vi "modbus asynch.vi"(11 "Modbus Module runtime in":refnum<class "Modbus Module runtime.lvclass">) -> (0 "error out":errorcluster)   [LabVIEW 2014, in "Modbus Module runtime.lvclass"]
uses:
  Modbus Module runtime.lvclass
  Modbus Module runtime.lvclass/Modbus Module runtime.ctl
  process state enum.ctl
  message to background process.ctl
  command enum.ctl
  <vilib>/NI/Tag Bus/table/data table.ctl
  response from background process.ctl
  response enum.ctl
  <vilib>/NI/Tag Bus/table/data table.lvlib
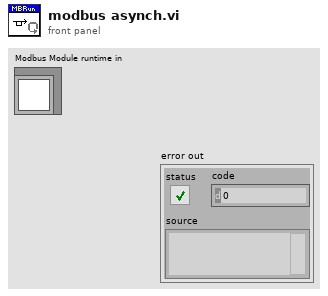
[diagram p1: front panel]
types:
  T1 = typedef "Modbus Module runtime.lvclass/response from background process.ctl" = cluster{"response enum":T2, "datapack":refnum<data-value>, "error code":i32}
  T2 = typedef "Modbus Module runtime.lvclass/response enum.ctl" = enum16{"exit", "return buffer", "error"}
  T3 = typedef "Modbus Module runtime.lvclass/message to background process.ctl" = cluster{"command enum":T4, "datapack":refnum<data-value>}
  T4 = typedef "Modbus Module runtime.lvclass/command enum.ctl" = enum16{"stop", "input", "output"}
  T5 = typedef "Modbus Module runtime.lvclass/process state enum.ctl" = enum16{"wait for message", "report error", "exit"}
  T6 = typedef "tag bus.lvlib/data table.lvlib/data table.ctl" = cluster{"Double":dbl[], "Single":sgl[], "I64":i64[], "I32":i32[], "I16":i16[], "I8":i8[], "U64":u64[], "U32":u32[], "U16":u16[], "U8":u8[], "Boolean":bool[], "String":string[], "Array of Double":cluster{"DBL Array":dbl[]}[], "Array of Single":cluster{"SGL Array":sgl[]}[], "Array of I64":cluster{"I64 Array":i64[]}[], "Array of I32":cluster{"I32 Array":i32[]}[], "Array of I16":cluster{"I16 Array":i16[]}[], "Array of I8":cluster{"I8 Array":i8[]}[], "Array of U64":cluster{"U64 Array":u64[]}[], "Array of U32":cluster{"U32 Array":u32[]}[], "Array of U16":cluster{"U16 Array":u16[]}[], "Array of U8":cluster{"U8 Array":u8[]}[], "Array of Boolean":cluster{"Boolean Array":bool[]}[], "Array of String":cluster{"String Array":string[]}[]}
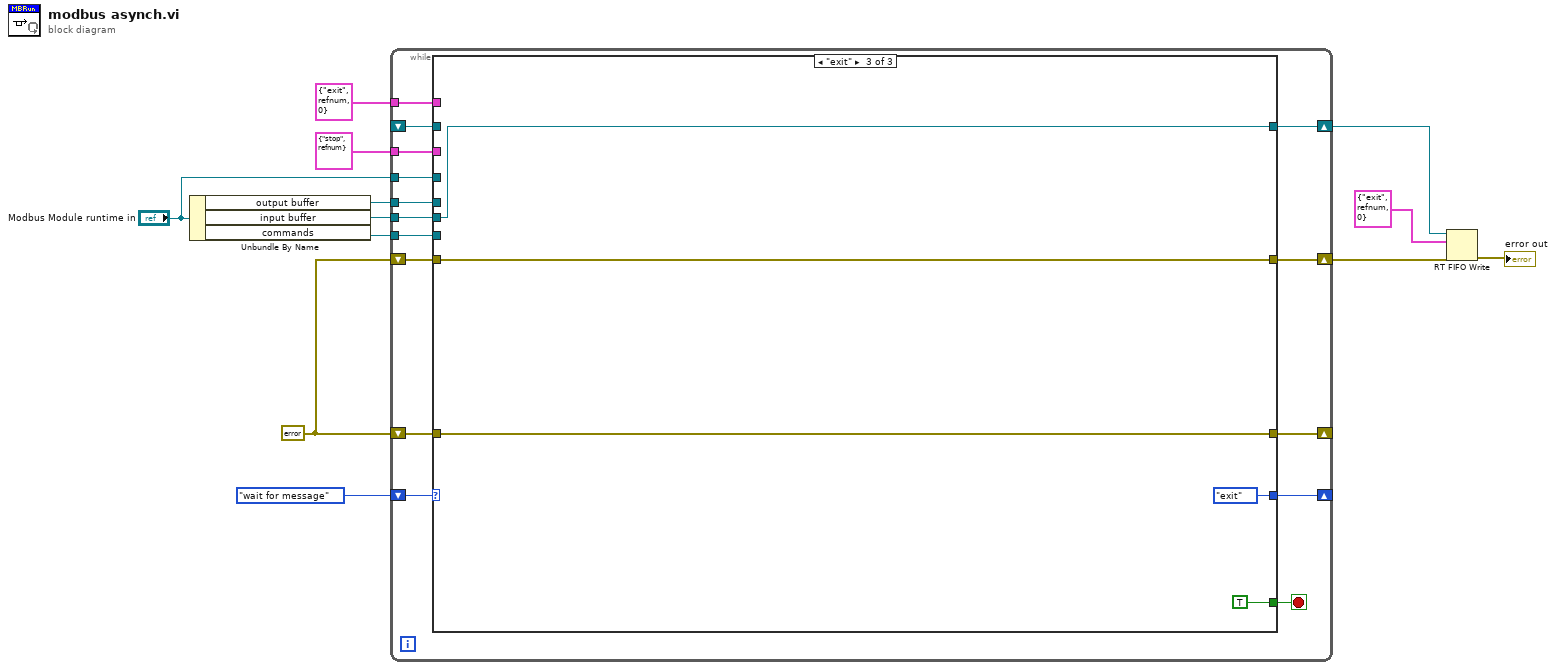
[diagram p0: block diagram]
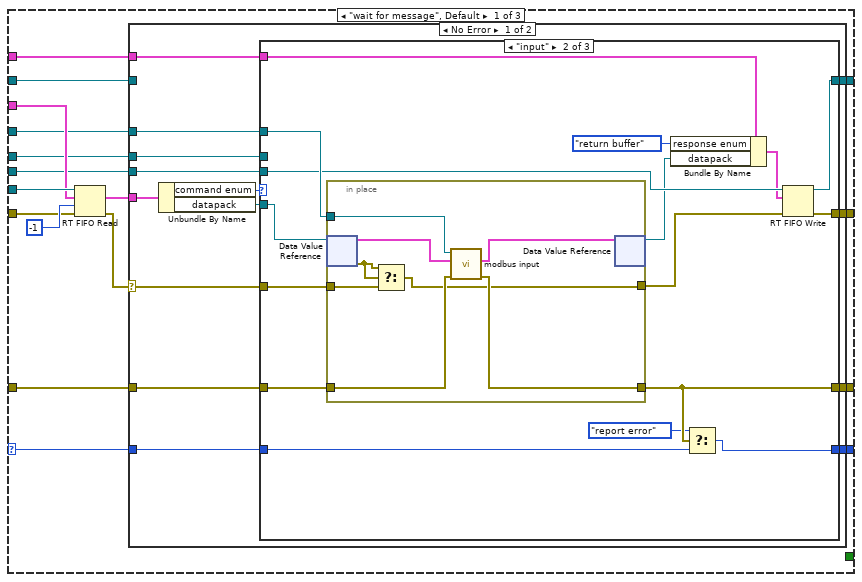
[diagram p2: hidden frame]
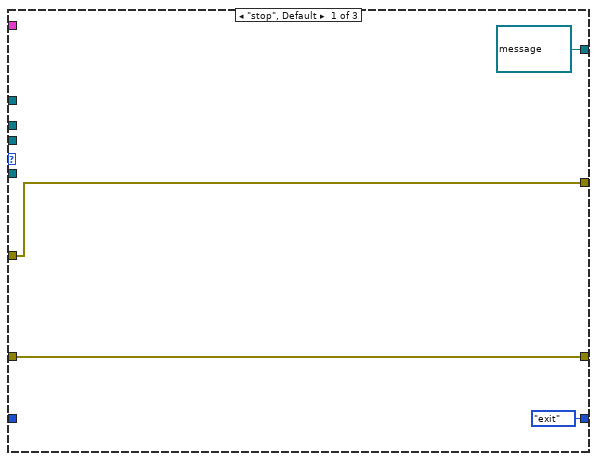
[diagram p3: hidden frame]
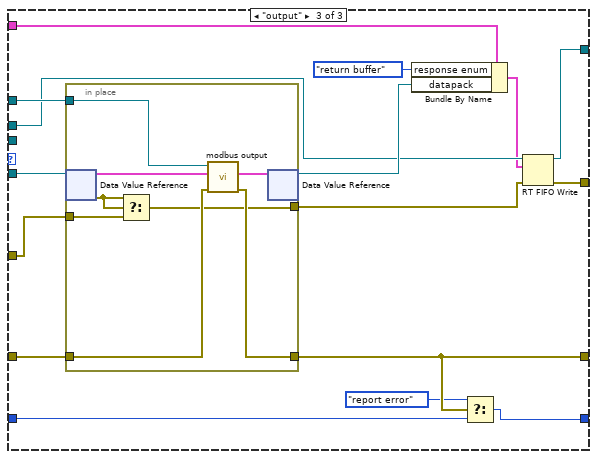
[diagram p4: hidden frame]
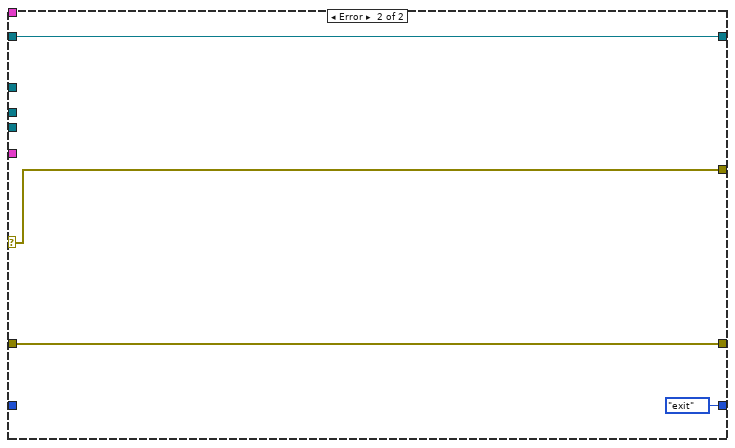
[diagram p5: hidden frame]
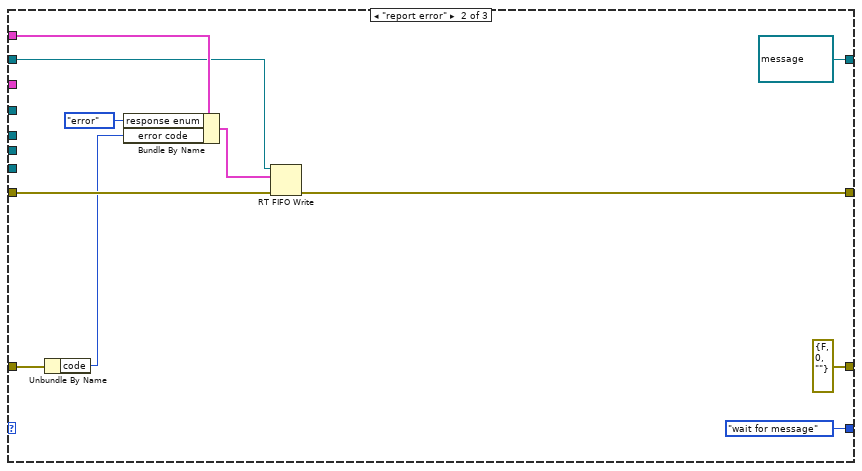
[diagram p6: hidden frame]
diagram:
  w7 = errorcluster {"status"=FALSE, "code"=0, "source"=""} ("error out")
  n1 = Unbundle By Name("Modbus Module runtime in") -> ("output buffer"=w5:refnum<k33>, "input buffer"=w8:refnum<k33>, "commands"=w11:refnum<k33>)
  n2 = while {
    shift-right: [w18] -> _
    shift-left: process_state_enum."wait for message" ("process state") -> [w27]
    tunnel: w11 -> [w26]
    tunnel: T3 {"command enum"=enum."stop", "datapack"=refnum} ("message") -> [w25]
    shift-right: [w21] -> w4
    shift-left: w7 -> [w24]
    tunnel: "Modbus Module runtime in" -> [w23]
    tunnel: w8 -> [w22]
    shift-right: [w19] -> _
    shift-left: w7 -> [w20]
    shift-right: [w16] -> w3
    shift-left: _ -> [w15]
    tunnel: T1 {"response enum"=enum."exit", "datapack"=refnum, "error code"=0} ("element") -> [w14]
    tunnel: w5 -> [w13]
    stop <- w17 stop-if-true
    n3 = case shown="\"exit\"" w27 {
      selector: w27 -> [w34 _ _]
      tunnel: w26 -> [w43 _ _]
      tunnel: w25 -> [w42 _ _]
      tunnel: w24 -> [w37 w125 w128]
      tunnel: w23 -> [w40 _ _]
      tunnel: w22 -> [w39 _ w126]
      tunnel: [w38 w118 w128] -> w21
      tunnel: w20 -> [w36 w122 w129]
      tunnel: [w35 errorcluster {"status"=FALSE, "code"=0, "source"=""} ("error out") w129] -> w19
      tunnel: [w33 process_state_enum."wait for message" ("process state") process_state_enum."exit" ("process state")] -> w18
      tunnel: [_ _ TRUE] -> w17
      tunnel: [w32 refnum<k33> refnum ("input buffer") w126] -> w16
      tunnel: w15 -> [w28 w121 _]
      tunnel: w14 -> [w31 w124 _]
      tunnel: w13 -> [w30 _ _]
      frame "wait for message", Default {
        n4 = RT FIFO Read(0:w43, 1:w42, 2:-1 ("timeout in ms (0)"), 3:w37) -> (9:w41:T3, 11:w29:errorcluster)  [unwired: 3 out]
        n5 = case shown="No Error" w29 {
          selector: w29 -> [w45 w111]
          tunnel: w41 -> [w58 _]
          tunnel: w40 -> [w55 _]
          tunnel: w39 -> [w54 _]
          tunnel: [w53 w111] -> w38
          tunnel: w36 -> [w52 w112]
          tunnel: [w51 w112] -> w35
          tunnel: w34 -> [w50 _]
          tunnel: [w49 process_state_enum."exit" ("process state")] -> w33
          tunnel: [w48 w114] -> w32
          tunnel: w31 -> [w47 _]
          tunnel: w30 -> [w46 _]
          tunnel: w28 -> [_ w114]
          frame No Error {
            n6 = Unbundle By Name(w58) -> ("command enum"=w57:T4, "datapack"=w56:refnum<data-value>)
            n7 = case shown="\"input\"" w57 {
              tunnel: w56 -> [_ w77 w102]
              tunnel: w55 -> [_ w78 w100]
              tunnel: w45 -> [w60 w76 w101]
              tunnel: w54 -> [_ w74 _]
              tunnel: [w60 w70 w87] -> w53
              tunnel: w52 -> [w61 w69 w99]
              tunnel: [w61 w68 w98] -> w51
              tunnel: w50 -> [_ w67 w97]
              tunnel: [process_state_enum."exit" ("process state") w65 w95] -> w49
              tunnel: [refnum<k33> refnum ("output buffer") w64 w88] -> w48
              tunnel: w47 -> [_ w63 w94]
              tunnel: w46 -> [_ _ w90]
              frame "stop", Default {
              }
              frame "input" {
                n8 = in-place {
                  in-place-border: w78 -> [w86]
                  in-place-border: w76 -> [w82]
                  in-place-border: [w79] -> w75
                  in-place-border: w69 -> [w81]
                  in-place-border: [w80] -> w68
                  n9 = in-place-dvr #1(w77) -> (w85:T6, w83:errorcluster)
                  n10 = Select(t=w83, s=w83, f=w82) -> (s? t:f=w79:errorcluster)
                  n11 = call-dynamic "modbus input.vi"("error in (no error)"=w81, "data table in"=w85, "Modbus Module runtime in"=w86) -> ("error out"=w80:errorcluster, "data table out"=w84:T6)  [unwired: 6 in, 1 out]
                  n12 = in-place-dvr #1(w84) -> (w72:refnum<data-value>)  [unwired: 1 out]
                }
                n13 = Bundle By Name(cluster=w63, "response enum"=response_enum."return buffer", "datapack"=w72) -> (w71:T1)
                n14 = Select(t=process_state_enum."report error", s=w68, f=w67) -> (s? t:f=w65:T5)
                n15 = RT FIFO Write(0:w74, 1:w71, 3:w75) -> (8:w64:refnum<k33>, 11:w70:errorcluster)  [unwired: 2 in, 2 out]
              }
              frame "output" {
                n16 = in-place {
                  in-place-border: w101 -> [w109]
                  in-place-border: w100 -> [w108]
                  in-place-border: w99 -> [w105]
                  in-place-border: [w104] -> w98
                  in-place-border: [w103] -> w91
                  n17 = in-place-dvr #2(w102) -> (w107:T6, w110:errorcluster)
                  n18 = Select(t=w110, s=w110, f=w109) -> (s? t:f=w103:errorcluster)
                  n19 = call-dynamic "modbus output.vi"("error in (no error)"=w105, "data table in"=w107, "Modbus Module runtime in"=w108) -> ("error out"=w104:errorcluster, "data table out"=w106:T6)  [unwired: 6 in, 1 out]
                  n20 = in-place-dvr #2(w106) -> (w92:refnum<data-value>)  [unwired: 1 out]
                }
                n21 = Bundle By Name(cluster=w94, "response enum"=response_enum."return buffer", "datapack"=w92) -> (w89:T1)
                n22 = Select(t=process_state_enum."report error", s=w98, f=w97) -> (s? t:f=w95:T5)
                n23 = RT FIFO Write(0:w90, 1:w89, 3:w91) -> (8:w88:refnum<k33>, 11:w87:errorcluster)  [unwired: 2 in, 2 out]
              }
            }
          }
          frame Error {
          }
        }
      }
      frame "report error" {
        n24 = Unbundle By Name(w122) -> ("code"=w115:i32)
        n25 = Bundle By Name(cluster=w124, "response enum"=response_enum."error", "error code"=w115) -> (w120:T1)
        n26 = RT FIFO Write(0:w121, 1:w120, 3:w125) -> (11:w118:errorcluster)  [unwired: 2 in, 3 out]
      }
      frame "exit" {
      }
    }
  }
  n27 = RT FIFO Write(0:w3, 1:T1 {"response enum"=enum."exit", "datapack"=refnum, "error code"=0} ("element"), 3:w4) -> (11:→"error out":errorcluster)  [unwired: 2 in, 3 out]
